vi "Image_Folder.vi"(8 "New":i32, 9 "Old":i32, 10 "Other":i32, 11 "input cluster":T1={"Pinch-valve"="Test Sample", "XLP 6000 Pump"="MRJ", "Camera1"="", "Camera2"="", "Img_Capt"=FALSE, "Actuator"=FALSE, "Pump"=FALSE, "Cam 1"=FALSE, "Cam 2"=FALSE, "Empty_Refill"=FALSE, "Crop"=FALSE, "Light intensity"=0, "Exposure Time"=0.0, "Sample Name"="", "Operator"="", "Calibration 1"=path "C:/Users/au540322/Desktop/IHS_Project/images/Debris/Debris_0/Debris_0_2019_06_01-23-32-49-686.PNG", "Calibration 2"=path "C:/Users/au540322/Desktop/IHS_Project/images/Debris/Debris_0/Debris_0_2019_06_01-23-32-49-686.PNG", "Framerate"=1, "Timeout Sample"=1, "Collection date"="", "Sample size threshold"=500, "Empty start"=500, "Command"="", "Station"="", "Species Name"="", "Other Notes"="", "Aperture"=enum."Item 3", "Image Process Queue Size"=100, "Image Save Queue Size"=0, "Overload threshold"=0, "Max Framerate"=0, "Rectangle 1"={"Left"=0, "Top"=0, "Right"=0, "Bottom"=0, "Rotation"=0.0}, "Rectangle 2"={"Left"=0, "Top"=100, "Right"=100, "Bottom"=0, "Rotation"=0.0}, "Detection Region %"=200.0, "Detect 1"=path "C:/Users/au540322/Desktop/IHS_Project/images/Debris/Debris_0/Debris_0_2019_06_01-23-32-49-686.PNG", "Detect 2"=path "C:/Users/au540322/Desktop/IHS_Project/images/Debris/Debris_0/Debris_0_2019_06_01-23-32-49-686.PNG", "Max large object threshold"=500, "Open(T)/Close(F)"=FALSE, "Img_Capt Begin"=FALSE, "Dispense Speed"=0, "Flush Size"=0, "Location"="", "Latitude"="", "Longitude"="", "Determiner"="", "Sex"="", "Camera1_Img"=refnum, "Camera2_Img"=refnum, "Img1_Orig_Disp"=refnum, "Img2_Orig_Disp"=refnum, "Img1_Orig_RGB"=refnum, "Img2_Orig_RGB"=refnum, "Blue_Plane_Extract"=refnum, "Subtracted_Plane"=refnum, "Img1_Binary"=refnum, "Img2_Binary"=refnum, "Crop_Mask"=refnum, "Img1_Save"=refnum, "Img2_Save"=refnum, "Img1_Cali_Full"=refnum, "Img2_Cali_Full"=refnum, "Img1_Cali_Detect"=refnum, "Img2_Cali_Detect"=refnum, "Cam 1 queue"=refnum, "Cam 2 queue"=refnum, "Cam 1 - save queue"=refnum, "Cam 2 - save queue"=refnum, "Overlay_Ring"=0, "SystemVersion"=0, "System Serial"="", "Legacy Cam Attributes"=FALSE, "Camera Orientation 1"="", "Camera Orientation 2"="", "Pixel to mm 1"=0.0, "Pixel to mm 2"=0.0, "CAM1 Model"=enum."a2A5328-15ucBAS", "CAM2 Model"=enum."a2A5328-15ucBAS"} {"SystemVersion" items=["Standard", "XL"]; "Overlay_Ring" items=["Session Data", "Extended Setup", "Buffer", "Camera", "Dispenser", "Stats", "Connections"]; "Flush Size" min=1; "Dispense Speed" min=1; "Rectangle 2"."Rotation" format="%.2f"; "Rectangle 2"."Left" scale=0.0..1024.0; "Rectangle 2"."Right" scale=0.0..1024.0; "Rectangle 1"."Rotation" format="%.2f"; "Rectangle 1"."Left" scale=0.0..1024.0; "Rectangle 1"."Right" scale=0.0..1024.0; "Max Framerate" min=1; "Overload threshold" min=1; "Image Save Queue Size" min=1; "Image Process Queue Size" min=1; "Empty start" min=1; "Sample size threshold" min=1; "Framerate" min=1; "Light intensity" scale=0.0..100.0}) -> (2 "Subfolder Name":string, 3 "Subfolder Path":string)   [LabVIEW 2022 SP3]
uses:
  controls/Data.ctl
  <vilib>/userdefined/High Color/IMAQdx.ctl
  <vilib>/vision/Image Controls.llb/IMAQ Image.ctl
panel:
  out "error out 2":errorcluster
  out "error out":errorcluster
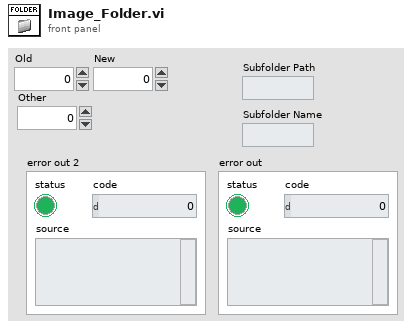
[diagram p1: front panel]
types:
  T1 = typedef "Data.ctl" = cluster{"Pinch-valve":refnum<visa-resource-name>, "XLP 6000 Pump":refnum<visa-resource-name>, "Camera1":T2, "Camera2":T2, "Img_Capt":bool, "Actuator":bool, "Pump":bool, "Cam 1":bool, "Cam 2":bool, "Empty_Refill":bool, "Crop":bool, "Light intensity":i32, "Exposure Time":dbl, "Sample Name":string, "Operator":string, "Calibration 1":path, "Calibration 2":path, "Framerate":i32, "Timeout Sample":i32, "Collection date":string, "Sample size threshold":i32, "Empty start":u32, "Command":string, "Station":string, "Species Name":string, "Other Notes":string, "Aperture":enum32{"Item 0", "Item 1", "Item 2", "Item 3"}, "Image Process Queue Size":i32, "Image Save Queue Size":i32, "Overload threshold":i32, "Max Framerate":i32, "Rectangle 1":T3, "Rectangle 2":T3, "Detection Region %":dbl, "Detect 1":path, "Detect 2":path, "Max large object threshold":i32, "Open(T)/Close(F)":bool, "Img_Capt Begin":bool, "Dispense Speed":i32, "Flush Size":i32, "Location":string, "Latitude":string, "Longitude":string, "Determiner":string, "Sex":string, "Camera1_Img":T4, "Camera2_Img":T4, "Img1_Orig_Disp":T4, "Img2_Orig_Disp":T4, "Img1_Orig_RGB":T4, "Img2_Orig_RGB":T4, "Blue_Plane_Extract":T4, "Subtracted_Plane":T4, "Img1_Binary":T4, "Img2_Binary":T4, "Crop_Mask":T4, "Img1_Save":T4, "Img2_Save":T4, "Img1_Cali_Full":T4, "Img2_Cali_Full":T4, "Img1_Cali_Detect":T4, "Img2_Cali_Detect":T4, "Cam 1 queue":refnum<queue>, "Cam 2 queue":refnum<queue>, "Cam 1 - save queue":refnum<queue>, "Cam 2 - save queue":refnum<queue>, "Overlay_Ring":u16, "SystemVersion":u16, "System Serial":string, "Legacy Cam Attributes":bool, "Camera Orientation 1":string, "Camera Orientation 2":string, "Pixel to mm 1":dbl, "Pixel to mm 2":dbl, "CAM1 Model":enum16{"a2A5328-15ucBAS", "acA1920-155uc"}, "CAM2 Model":enum16{"a2A5328-15ucBAS", "acA1920-155uc"}}
  T2 = typedef "IMAQdx.ctl" = refnum<k21>
  T3 = typedef "IMAQ Rectangle" = cluster{"Left":i32, "Top":i32, "Right":i32, "Bottom":i32, "Rotation":dbl}
  T4 = typedef "IMAQ Image.ctl" = refnum<image>
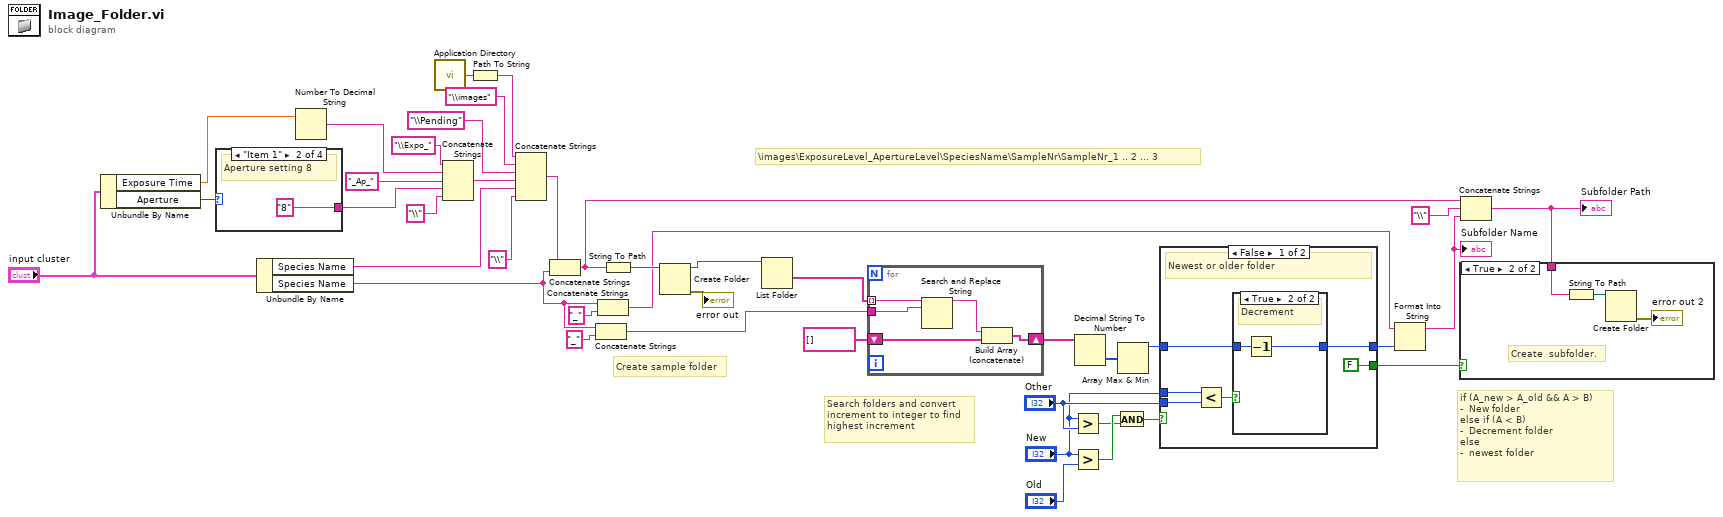
[diagram p0: block diagram]
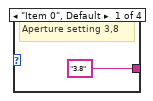
[diagram p2: hidden frame]
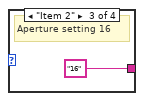
[diagram p3: hidden frame]
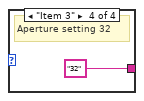
[diagram p4: hidden frame]
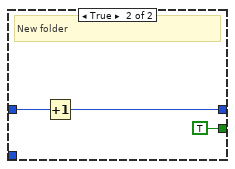
[diagram p6: hidden frame]
diagram:
  # "\\images\\ExposureLevel_ApertureLevel\\SpeciesName\\SampleNr\\SampleNr_1 .. 2 ... 3"
  # "if (A_new > A_old && A > B)\n-  New folder\nelse if (A < B)\n-  Decrement folder\nelse \n-  newest folder"
  # "Search folders and convert \nincrement to integer to find\nhighest increment"
  # "Create sample folder"
  n1 = Unbundle By Name("input cluster") -> ("Exposure Time"=w13:dbl, "Aperture"=w10:enum32{"Item 0", "Item 1", "Item 2", "Item 3"})
  n2 = case shown="\"Item 1\"" w10 {
    tunnel: ["3.8" "8" "16" "32"] -> w7
    frame "Item 0", Default {
      # "Aperture setting 3,8"
    }
    frame "Item 1" {
      # "Aperture setting 8"
    }
    frame "Item 2" {
      # "Aperture setting 16"
    }
    frame "Item 3" {
      # "Aperture setting 32"
    }
  }
  n3 = Unbundle By Name("input cluster") -> ("Species Name"=w18:string, "Species Name"=w16:string)
  n4 = Number To Decimal String(number=w13) -> (decimal integer string=w8:string)  [unwired: 1 in]
  n5 = call <vilib>:"Application Directory.vi"() -> ("Application Directory"=w36:path)
  n6 = Concatenate Strings("\\Expo_" ("string"), w8, "_Ap_" ("string"), w7, "\\" ("string")) -> (w5:string)
  n7 = Path To String(path=w36) -> (string=w3:string)
  n8 = Concatenate Strings(w3, "\\images" ("string"), "\\Pending" ("string"), w5, w18, "\\" ("string")) -> (w17:string)
  n9 = Concatenate Strings(w17, w16) -> (w15:string)
  n10 = Concatenate Strings(w16, "_" ("string")) -> (w34:string)
  n11 = Concatenate Strings(w16, "_" ("string")) -> (w4:string)
  n12 = String To Path(string=w15) -> (path=w37:path)
  n13 = Create Folder(path (use dialog)=w37) -> (created path=w40:path, error out=→"error out":errorcluster)  [unwired: 2 in, 1 out]
  n14 = List Folder(path=w40) -> (folder names=w35:string[])  [unwired: 3 in, 3 out]
  n15 = for {
    tunnel: w35 -> [w50] mode=indexing
    tunnel: w34 -> [w49]
    shift-right: [w47] -> w32
    shift-left: string[] [] -> [w46]
    n16 = Search and Replace String(input string=w50, search string=w49) -> (result string=w48:string)  [unwired: 6 in, 3 out]
    n17 = Build Array (concatenate)(w48, w46) -> (w47:string[])
  }
  n18 = Greater?(x="New", y="Other") -> (0:w26:bool)
  n19 = Greater?(x="New", y="Old") -> (0:w27:bool)
  n20 = Decimal String To Number(string=w32) -> (number=w31:i32[])  [unwired: 2 in, 1 out]
  n21 = And(x=w27, y=w26) -> (x .and. y?=w25:bool)
  n22 = Array Max & Min(array=w31) -> (max value=w21:i32)  [unwired: 3 out]
  n23 = case shown="False" w25 {
    tunnel: "Other" -> [w56 _]
    tunnel: "New" -> [w55 _]
    tunnel: [FALSE ("New sample (F)") TRUE ("New sample (F)")] -> w22
    tunnel: w21 -> [w53 w61]
    tunnel: [w52 w60] -> w20
    frame False {
      # "Newest or older folder"
      n24 = Less?(x=w55, y=w56) -> (x < y?=w54:bool)
      n25 = case shown="True" w54 {
        tunnel: w53 -> [w57 w59]
        tunnel: [w57 w58] -> w52
        frame False {
          # "Newest folder"
        }
        frame True {
          # "Decrement"
          n26 = Decrement(x=w59) -> (x-1=w58:i32)
        }
      }
    }
    frame True {
      # "New folder"
      n27 = Increment(x=w61) -> (x+1=w60:i32)
    }
  }
  n28 = Format Into String(initial string=w4, w20) -> (resulting string=w29:string)  [unwired: 2 in, 1 out]
  "Subfolder Name" <- w29
  n29 = Concatenate Strings(w15, "\\" ("string"), w29) -> (w19:string)
  "Subfolder Path" <- w19
  n30 = case shown="True" w22 {
    tunnel: w19 -> [_ w63]
    frame False {
    }
    frame True {
      # "Create  subfolder."
      n31 = String To Path(string=w63) -> (path=w64:path)
      n32 = Create Folder(path (use dialog)=w64) -> (error out=→"error out 2":errorcluster)  [unwired: 2 in, 2 out]
    }
  }
